vi "toGPS-Epoch.vi"(11 "Epoch in":refnum<class "Epoch.lvclass">) -> (2 "GPS Epoch Time":i64, 3 "Epoch":refnum<class "Epoch.lvclass">)   [LabVIEW 2013, in "Epoch.lvclass"]
uses:
  Epoch.lvclass
  Epoch.lvclass/Epoch.ctl
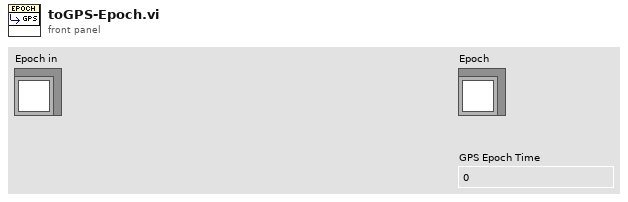
[diagram p1: front panel]
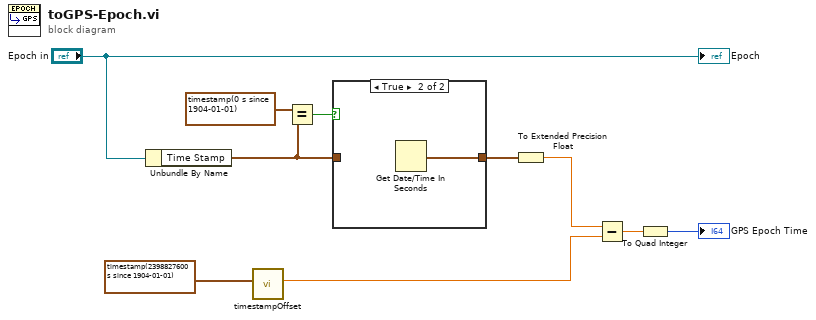
[diagram p0: block diagram]
diagram:
  n1 = Unbundle By Name("Epoch in") -> ("Time Stamp"=w1:timestamp)
  n2 = call "timestampOffset.vi"("Reference Time"=timestamp(2398827600 s since 1904-01-01) ("Timestamp")) -> ("Timestamp Offset"=w5:ext)  [unwired: 10 in]
  n3 = Equal?(x=timestamp(0 s since 1904-01-01), y=w1) -> (x = y?=w3:bool)
  n4 = case shown="True" w3 {
    tunnel: [w11 w12] -> w2
    tunnel: w1 -> [w11 _]
    frame False {
    }
    frame True {
      n5 = Get Date/Time In Seconds() -> (seconds since 1Jan1904=w12:timestamp)
    }
  }
  n6 = To Extended Precision Float(1:w2) -> (0:w7:ext)
  n7 = Subtract(x=w7, y=w5) -> (x-y=w9:ext)
  n8 = To Quad Integer(1:w9) -> (0:→"GPS Epoch Time":i64)
  "Epoch" <- "Epoch in"
